vi "SPI Simple.vi"() -> ()   [LabVIEW 2021]
panel:
  in  "# Bytes To Transfer (1-50)":i32=4 min=1 max=50
  out "U8 Array Read":u8[](array[numeric])
  in  "U8 Array Write":u8[](array[numeric])=[170, 240, 170, 240]
  out "Error Message":string
  out "error out":errorcluster
  # "Simple SPI example uses the first found USB device.  You can short MOSI to MISO for testing.  Does\na single SPI call, so limited to 1-50 bytes of data transfer.\n\nMOSI    FIO2\nMISO    FIO3\nCLK      FIO0\nCS        FIO1\n\nIf you short MISO to MOSI, then you will read back the same bytes that you write.  If you short\nMISO to GND, then you will read back zeros.  If you short MISO to VS or leave it\nunconnected, you will read back 255s.\n\nTested with UD V2.77, U3 firmware V1.44, and UE9 firmware 1.40/1.84 (Comm/Control).  Will\nhave to change to FIO4-7 on a U3-HV."
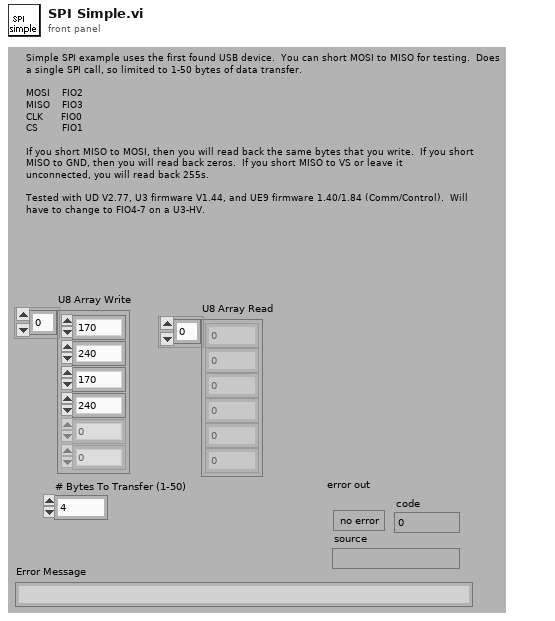
[diagram p1: front panel]
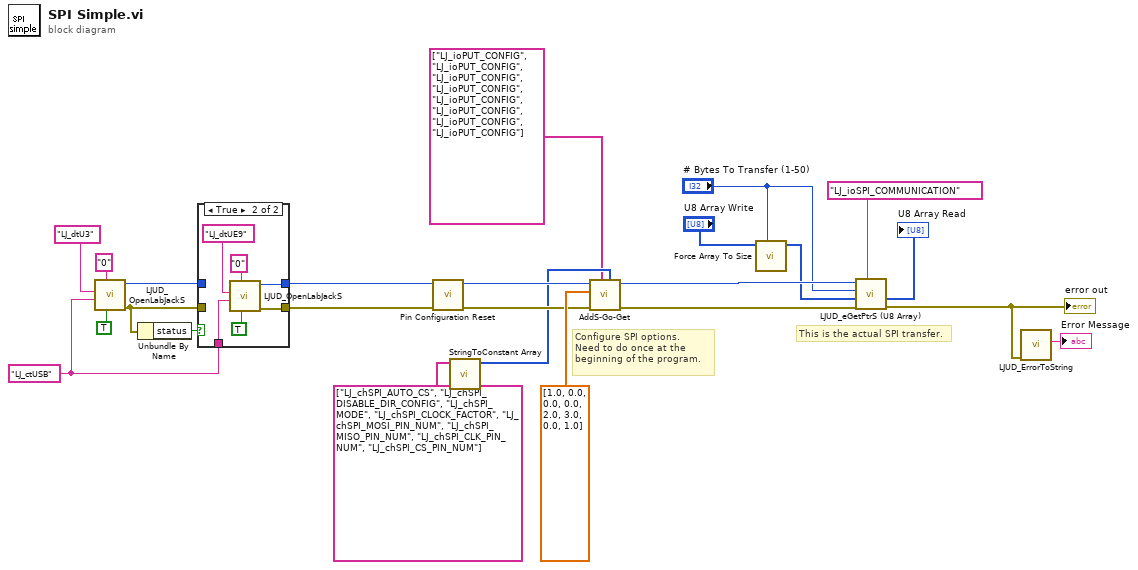
[diagram p0: block diagram]
diagram:
  w3 = "LJ_ctUSB" ("ConnectionType")
  # "This is the actual SPI transfer."
  # "Configure SPI options.\nNeed to do once at the\nbeginning of the program."
  n1 = call "LJUD_OpenLabJackS.vi"("FirstFound"=TRUE, "Address"="0", "ConnectionType"=w3, "DeviceType"="LJ_dtU3") -> ("error out"=w7:errorcluster, "Handle"=w5:i32)  [unwired: 5 in, 1 out]
  n2 = Unbundle By Name(w7) -> ("status"=w8:bool)
  n3 = case shown="True" w8 {
    tunnel: w7 -> [w26 _]
    tunnel: [w26 w29] -> w6
    tunnel: w5 -> [w25 _]
    tunnel: [w25 w28] -> w4
    tunnel: w3 -> [_ w30]
    frame False {
    }
    frame True {
      n4 = call "LJUD_OpenLabJackS.vi"("FirstFound"=TRUE, "Address"="0", "ConnectionType"=w30, "DeviceType"="LJ_dtUE9") -> ("error out"=w29:errorcluster, "Handle"=w28:i32)  [unwired: 5 in, 1 out]
    }
  }
  n5 = call "Pin Configuration Reset.vi"("error in"=w6, "Handle In"=w4) -> ("error out"=w10:errorcluster, "Handle Out"=w9:i32)  [unwired: 8 in]
  n6 = call "StringToConstant Array.vi"("String Constant Array In"=string[] ["LJ_chSPI_AUTO_CS", "LJ_chSPI_DISABLE_DIR_CONFIG", "LJ_chSPI_MODE", "LJ_chSPI_CLOCK_FACTOR", "LJ_chSPI_MOSI_PIN_NUM", "LJ_chSPI_MISO_PIN_NUM", "LJ_chSPI_CLK_PIN_NUM", "LJ_chSPI_CS_PIN_NUM"] ("IOTypes")) -> ("I32 Constant Array Out"=w2:i32[])  [unwired: 10 in]
  n7 = call "AddS-Go-Get.vi"("Channels"=w2, "IOTypes"=string[] ["LJ_ioPUT_CONFIG", "LJ_ioPUT_CONFIG", "LJ_ioPUT_CONFIG", "LJ_ioPUT_CONFIG", "LJ_ioPUT_CONFIG", "LJ_ioPUT_CONFIG", "LJ_ioPUT_CONFIG", "LJ_ioPUT_CONFIG"], "error in"=w10, "Values Write"=dbl[] [1.0, 0.0, 0.0, 0.0, 2.0, 3.0, 0.0, 1.0], "Handle In"=w9) -> ("error out"=w15:errorcluster, "Handle Out"=w14:i32)  [unwired: 4 in, 1 out]
  n8 = call "Force Array To Size.vi"("# Elements"="# Bytes To Transfer (1-50)", "I32 Array In"="U8 Array Write") -> ("I32 Array Out"=w11:i32[])  [unwired: 6 in, 3 out]
  n9 = call "LJUD_eGetPtrS (U8 Array).vi"("IOType"="LJ_ioSPI_COMMUNICATION", "error in"=w15, "U8 Array Write"=w11, "Value"="# Bytes To Transfer (1-50)", "Handle In"=w14) -> ("error out"=w22:errorcluster, "U8 Array Read"=→"U8 Array Read":u8[])  [unwired: 3 in, 2 out]
  "error out" <- w22
  n10 = call "LJUD_ErrorToString.vi"("error in"=w22) -> ("String"=→"Error Message":string)  [unwired: 10 in]
